vi "Get MetaData from Results.vi"(8 "error in":errorcluster, 10 "MeasurementPluginService in":refnum<class "MeasurementPluginService.lvclass">, 11 "Configuration Cluster":variant) -> (0 "error out":errorcluster, 2 "MeasurementPluginService out":refnum<class "MeasurementPluginService.lvclass">, 3 "outputs":T1[](array[typedef]))   [LabVIEW 2020, in "MeasurementLink Measurement Server.lvlib"]
uses:
  MeasurementLink Measurement Server.lvlib
  TypeDefs/OutputParameter.ctl
  TypeDefs/Parameter_AnnotationsEntry.ctl
  Classes/MeasurementPluginService/MeasurementPluginService.lvclass
  <vilib>/Utility/Data Type/NI_Data Type.lvlib
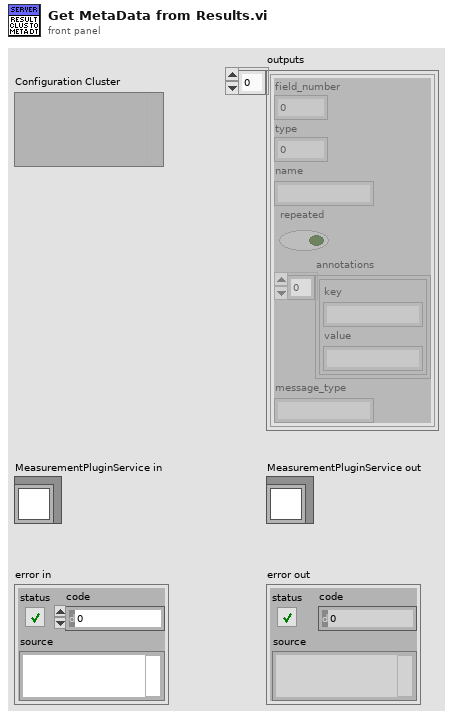
[diagram p1: front panel]
types:
  T1 = typedef "MeasurementLink Measurement Server.lvlib/OutputParameter.ctl" = cluster{"field_number":i32, "type":i32, "name":string, "repeated":bool, "annotations":T2[], "message_type":string}
  T2 = typedef "MeasurementLink Measurement Server.lvlib/Parameter_AnnotationsEntry.ctl" = cluster{"key":string, "value":string}
  T3 = typedef "MeasurementLink Measurement Server.lvlib/MeasurementPluginService.lvclass/Plugin Paths.ctl" = cluster{"Get Measurement Details VI Path":path, "Get Type Specializations VI Path":path, "Get UI Details VI Path":path, "Measurement Logic VI Path":path, "Measurement Configuration CTL Path":path, "Measurement Results CTL Path":path}
  T4 = cluster{"Parameter Name":string, "Annotations":T2[]}[]
  T5 = typedef "MeasurementLink Measurement Server.lvlib/google_protobuf_Field_Kind.ctl" = enum32{"TYPE_UNKNOWN", "TYPE_DOUBLE", "TYPE_FLOAT", "TYPE_INT64", "TYPE_UINT64", "TYPE_INT32", "TYPE_FIXED64", "TYPE_FIXED32", "TYPE_BOOL", "TYPE_STRING", "TYPE_GROUP", "TYPE_MESSAGE", "TYPE_BYTES", "TYPE_UINT32", "TYPE_ENUM", "TYPE_SFIXED32", "TYPE_SFIXED64", "TYPE_SINT32", "TYPE_SINT64"}
  T6 = typedef "NI_Data Type.lvlib/Data Type.ctl" = enum8{"Invalid Type", "Void", "I8", "I16", "I32", "I64", "U8", "U16", "U32", "U64", "Single Float", "Double Float", "Extended Float", "Single Complex", "Double Complex", "Extended Complex", "Enum U8", "Enum U16", "Enum U32", "Enum U64", "Single Float With Unit", "Double Float With Unit", "Extended Float With Unit", "Single Complex with Unit", "Double Complex with Unit", "Extended Complex with Unit", "Boolean", "String", "Path", "Picture", "Tag", "Array", "Cluster", "Variant", "LV Variant", "Waveform", "Timestamp", "Digital Waveform", "Digital Data", "ExpressData", "Refnum", "External Data", "VI", "Poly VI", "LabVIEW Class Instance", "Fixed Point", "Set Collection", "Map Collection"}
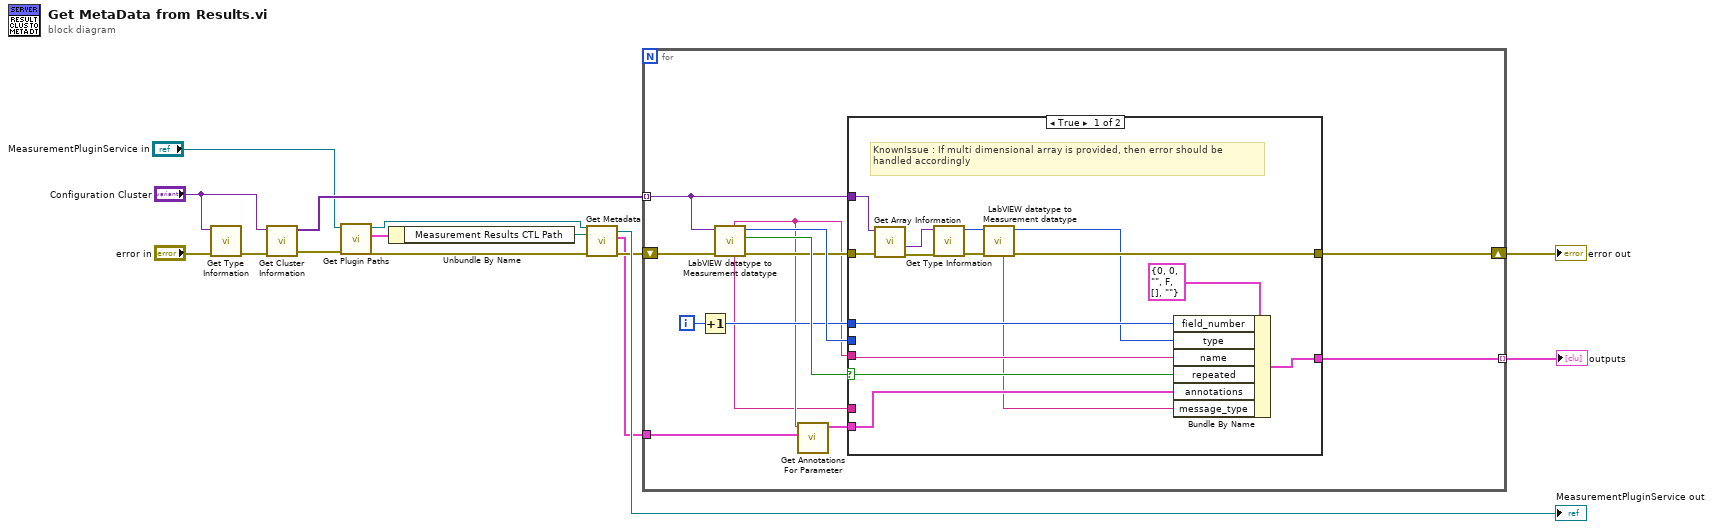
[diagram p0: block diagram]
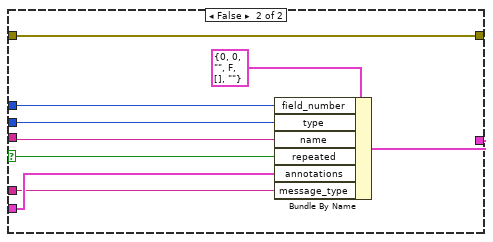
[diagram p2: hidden frame]
diagram:
  n1 = call <vilib>:"Get Type Information.vi"("error in (no error)"="error in", "variant"="Configuration Cluster") -> ("error out"=w15:errorcluster)  [unwired: 5 in, 4 out]
  n2 = call <vilib>:"Get Cluster Information.vi"("error in (no error)"=w15, "variant"="Configuration Cluster") -> ("error out"=w3:errorcluster, "cluster elements"=w14:variant[])  [unwired: 8 in]
  n3 = call-dynamic "Get Plugin Paths.vi"("error in (no error)"=w3, "MeasurementPluginService in"="MeasurementPluginService in") -> ("error out"=w6:errorcluster, "Plugin Paths"=w10:T3, "MeasurementPluginService out"=w2:refnum<class "MeasurementPluginService.lvclass">)  [unwired: 7 in]
  n4 = Unbundle By Name(w10) -> ("Measurement Results CTL Path"=w9:path)
  n5 = call "Get Metadata.vi"("error in (no error)"=w6, "measurement control path"=w9, "MeasurementPluginService in"=w2) -> ("error out"=w7:errorcluster, "Metadata Value"=w4:T4, "MeasurementPluginService out"=→"MeasurementPluginService out":refnum<class "MeasurementPluginService.lvclass">)  [unwired: 5 in]
  n6 = for {
    tunnel: w14 -> [w19] mode=indexing
    tunnel: [w25] -> w13 mode=indexing
    shift-right: [w22] -> w1
    shift-left: w7 -> [w18]
    tunnel: w4 -> [w20]
    i -> [w28]
    n7 = Increment(x=w28) -> (x+1=w23:i32)
    n8 = call "LabVIEW datatype to Measurement datatype.vi"("error in"=w18, "variant"=w19) -> ("error out"=w24:errorcluster, "array?"=w26:bool, "grpc_type"=w27:T5, "message_type"=w16:string, "name"=w17:string)  [unwired: 4 in, 1 out]
    n9 = call "Get Annotations For Parameter.vi"("Metadata Value"=w20, "Parameter Name"=w17) -> ("Annotations"=w21:T2[])  [unwired: 9 in]
    n10 = case shown="True" w26 {
      selector: w26 -> [w43 w52]
      tunnel: w23 -> [w35 w49]
      tunnel: w27 -> [_ w47]
      tunnel: [w30 w51] -> w25
      tunnel: w24 -> [w42 w50]
      tunnel: w19 -> [w41 _]
      tunnel: [w37 w50] -> w22
      tunnel: w17 -> [w33 w48]
      tunnel: w21 -> [w32 w46]
      tunnel: w16 -> [_ w44]
      frame True {
        # "KnownIssue : If multi dimensional array is provided, then error should be handled accordingly"
        n11 = call <vilib>:"Get Array Information.vi"("error in (no error)"=w42, "variant"=w41) -> ("error out"=w40:errorcluster, "array element data type"=w36:variant)  [unwired: 6 in, 2 out]
        n12 = call <vilib>:"Get Type Information.vi"("error in (no error)"=w40, "variant"=w36) -> ("error out"=w38:errorcluster, "type"=w39:T6)  [unwired: 5 in, 3 out]
        n13 = call "LabVIEW datatype to Measurement datatype.vi"("error in"=w38, "variant"=w39) -> ("error out"=w37:errorcluster, "grpc_type"=w34:T5, "message_type"=w29:string)  [unwired: 4 in, 3 out]
        n14 = Bundle By Name(cluster=T1 {"field_number"=0, "type"=0, "name"="", "repeated"=FALSE, "annotations"=[], "message_type"=""} ("OutputParameter"), "field_number"=w35, "type"=w34, "name"=w33, "repeated"=w43, "annotations"=w32, "message_type"=w29) -> (w30:T1)
      }
      frame False {
        n15 = Bundle By Name(cluster=T1 {"field_number"=0, "type"=0, "name"="", "repeated"=FALSE, "annotations"=[], "message_type"=""} ("OutputParameter"), "field_number"=w49, "type"=w47, "name"=w48, "repeated"=w52, "annotations"=w46, "message_type"=w44) -> (w51:T1)
      }
    }
  }
  "error out" <- w1
  "outputs" <- w13
